vi "报警信息.vi"(8 "error in (no error)":errorcluster, 11 "data in":T1) -> (0 "error out":errorcluster)   [LabVIEW 2016, in "超标留样集成.lvlib" / "ESTD1200.lvlib"]
uses:
  ESTD1200.lvlib
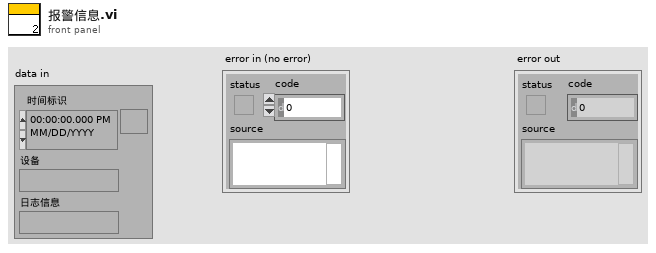
[diagram p1: front panel]
types:
  T1 = cluster{"时间标识":timestamp, "设备":string, "日志信息":string}
  T2 = typedef "报警信息字段定义.ctl" = cluster{"时间":timestamp, "参数":string, "元器件":string, "故障现象":string, "故障分析":string, "state":string, "code":string, "platform_alarm_code":string, "是否上报":string}
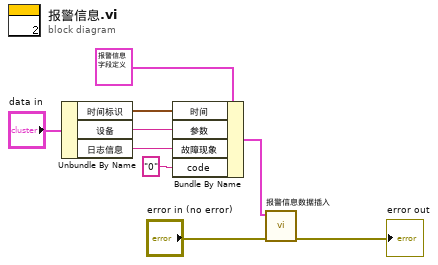
[diagram p0: block diagram]
diagram:
  n1 = Unbundle By Name("data in") -> ("时间标识"=w8:timestamp, "设备"=w7:string, "日志信息"=w6:string)
  n2 = Bundle By Name(cluster=T2 {"时间"=timestamp(0 s since 1904-01-01), "参数"="水样测试", "元器件"="N", "故障现象"="", "故障分析"="", "state"="", "code"="", "platform_alarm_code"="", "是否上报"=""} ("data"), "时间"=w8, "参数"=w7, "故障现象"=w6, "code"="0") -> (w5:T2)
  n3 = call "报警信息数据插入.vi"("data"=w5, "错误输入（无错误）"="error in (no error)") -> ("错误输出"=→"error out":errorcluster)  [unwired: 8 in]
